vi "FGV_PSP - Mercury Actions.vi"(4 "error in":errorcluster, 6 "Function":enum16{"write", "read"}(ring), 7 "Actions":T1) -> (0 "error out":errorcluster, 3 "Actions":T1)   [LabVIEW 2016]
uses:
  Mercury - Typedefs/Actions.ctl
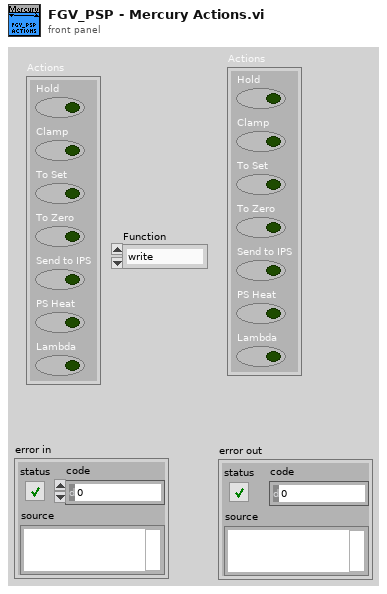
[diagram p1: front panel]
types:
  T1 = typedef "Actions.ctl" = cluster{"Hold":bool, "Clamp":bool, "To Set":bool, "To Zero":bool, "Send to IPS":bool, "PS Heat":bool, "Lambda":bool}
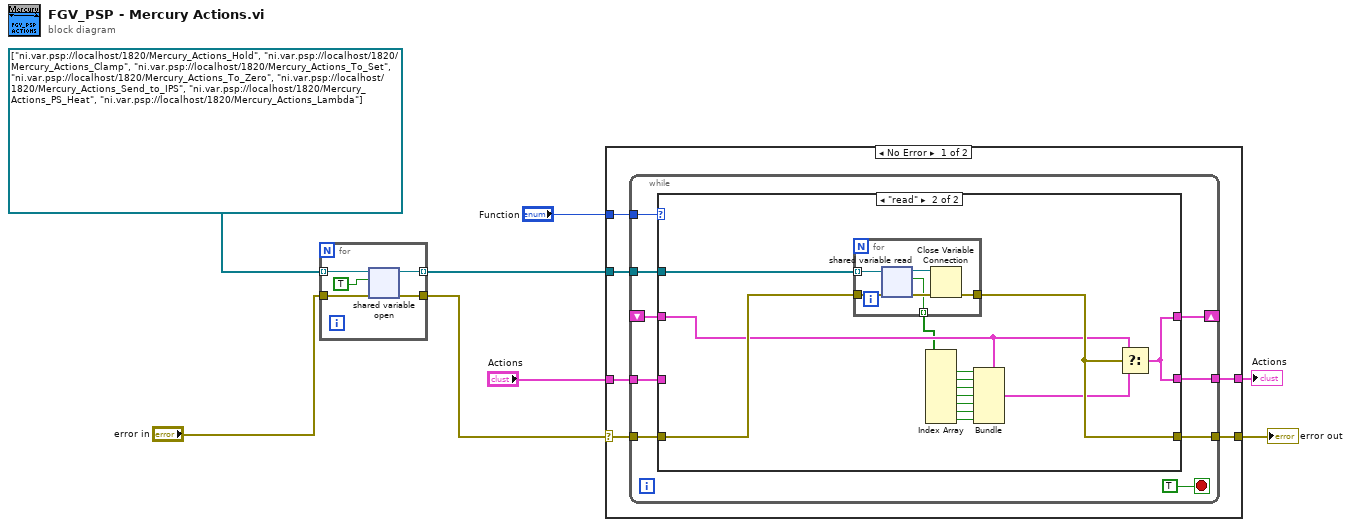
[diagram p0: block diagram]
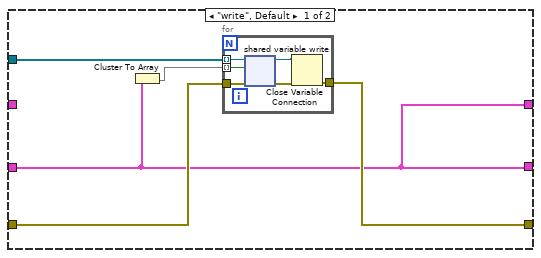
[diagram p2: hidden frame]
diagram:
  n1 = for {
    tunnel: [w13] -> w6 mode=indexing
    tunnel: [w12] -> w5
    tunnel: "error in" -> [w11]
    tunnel: refnum<k21>[] ["ni.var.psp://localhost/1820/Mercury_Actions_Hold", "ni.var.psp://localhost/1820/Mercury_Actions_Clamp", "ni.var.psp://localhost/1820/Mercury_Actions_To_Set", "ni.var.psp://localhost/1820/Mercury_Actions_To_Zero", "ni.var.psp://localhost/1820/Mercury_Actions_Send_to_IPS", "ni.var.psp://localhost/1820/Mercury_Actions_PS_Heat", "ni.var.psp://localhost/1820/Mercury_Actions_Lambda"] -> [w9] mode=indexing
    n2 = shared-variable-open(w9, w11, TRUE) -> (w13:refnum<k21>, w12:errorcluster)  [unwired: 1 in]
  }
  n3 = case shown="No Error" w5 {
    selector: w5 -> [w19 w61]
    tunnel: [w18 w61] -> w8
    tunnel: [w17 w60] -> w1
    tunnel: "Function" -> [w16 _]
    tunnel: w6 -> [w15 _]
    tunnel: "Actions" -> [w14 w60]
    frame No Error {
      n4 = while {
        shift-right: [w23] -> _
        shift-left: _ -> [w22]
        tunnel: w19 -> [w27]
        tunnel: [w26] -> w18
        tunnel: [w25] -> w17
        tunnel: w16 -> [w24]
        tunnel: w15 -> [w21]
        tunnel: w14 -> [w20]
        stop <- TRUE stop-if-true
        n5 = case shown="\"read\"" w24 {
          tunnel: w27 -> [w32 w51]
          tunnel: [w33 w50] -> w26
          tunnel: [w29 w53] -> w25
          tunnel: [w29 w53] -> w23
          tunnel: w22 -> [_ w49]
          tunnel: w21 -> [w31 w52]
          tunnel: w20 -> [w29 _]
          frame "write", Default {
            n6 = Cluster To Array(cluster=w29) -> (array=w30:bool[])
            n7 = for {
              tunnel: [w38] -> w33
              tunnel: w32 -> [w36]
              tunnel: w31 -> [w35] mode=indexing
              tunnel: w30 -> [w34] mode=indexing
              n8 = shared-variable-write(w35, w36, w34) -> (w37:refnum<k21>, w39:errorcluster)
              n9 = Close Variable Connection(8:w39, 11:w37) -> (0:w38:errorcluster)
            }
          }
          frame "read" {
            n10 = for {
              tunnel: [w57] -> w50
              tunnel: w52 -> [w56] mode=indexing
              tunnel: w51 -> [w55]
              tunnel: [w54] -> w47 mode=indexing
              n11 = shared-variable-read(w56, w55) -> (w59:refnum<k21>, w58:errorcluster, w54:bool)  [unwired: 1 out]
              n12 = Close Variable Connection(8:w58, 11:w59) -> (0:w57:errorcluster)
            }
            n13 = Index Array(array=w47) -> (element #1=w46:bool, element #2=w45:bool, element #3=w44:bool, element #4=w43:bool, element #5=w42:bool, element #6=w41:bool, element #7=w40:bool)  [unwired: 7 in]
            n14 = Bundle(cluster=w49, "Hold"=w46, "Clamp"=w45, "To Set"=w44, "To Zero"=w43, "Send to IPS"=w42, "PS Heat"=w41, "Lambda"=w40) -> (w48:T1)
            n15 = Select(t=w49, s=w50, f=w48) -> (s? t:f=w53:T1)
          }
        }
      }
    }
    frame Error {
    }
  }
  "error out" <- w8
  "Actions" <- w1
